vi "SetAngles.vi"(8 "error in (no error)":errorcluster, 10 "Angles":T1, 11 "reference in":refnum<class "Manipulator.lvclass">) -> (0 "error out":errorcluster, 3 "reference out":refnum<class "Manipulator.lvclass">)   [LabVIEW 2014, in "Manipulator.lvclass"]
uses:
  Manipulator.lvclass
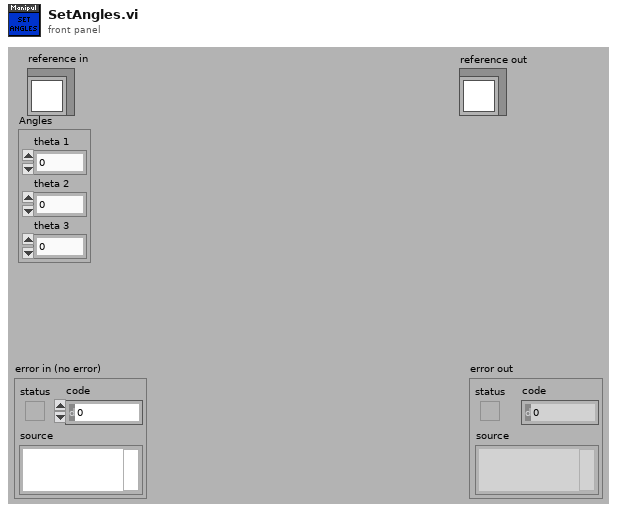
[diagram p1: front panel]
types:
  T1 = cluster{"theta 1":dbl, "theta 2":dbl, "theta 3":dbl}
  T2 = typedef "Manipulator.lvclass/ObjectAttributes.ctl" = cluster{"Coordinates":cluster{"X":dbl, "Y":dbl, "Z":dbl}, "Angles":cluster{"THETA_1":dbl, "THETA_2":dbl, "THETA_3":dbl, "THETA_4":dbl, "THETA_5":dbl, "THETA_6":dbl, "THETA_7":dbl, "THETA_8":dbl, "THETA_9":dbl, "THETA_10":dbl}, "Lengths":cluster{"a":dbl, "b":dbl, "c":dbl, "d":dbl, "e":dbl}, "Coordinates of joints":cluster{"A":cluster{"X":dbl, "Y":dbl, "Z":dbl}, "B":cluster{"X":dbl, "Y":dbl, "Z":dbl}, "C":cluster{"X":dbl, "Y":dbl, "Z":dbl}, "D":cluster{"X":dbl, "Y":dbl, "Z":dbl}}}
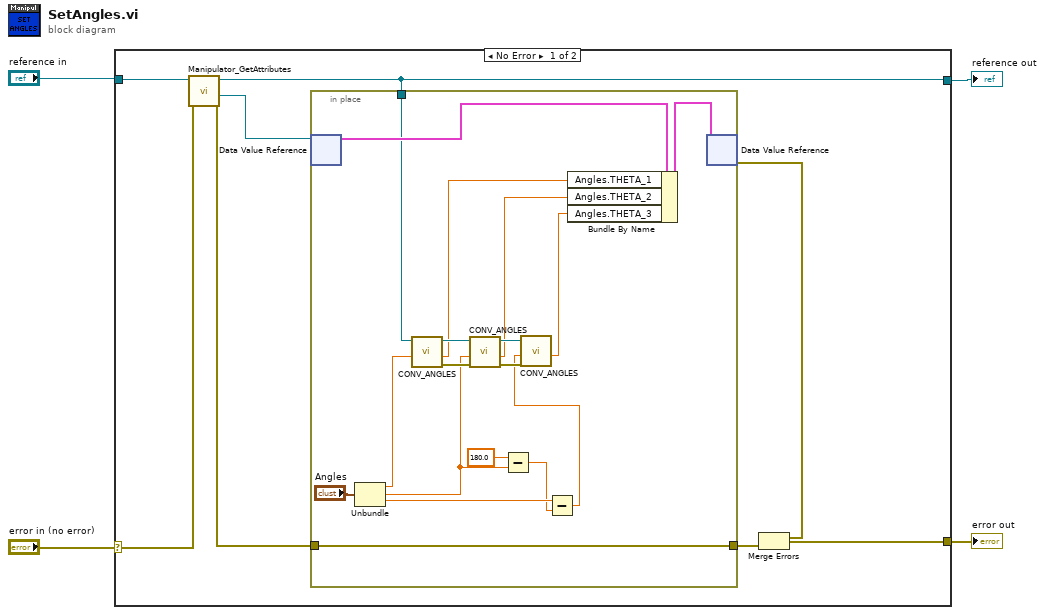
[diagram p0: block diagram]
diagram:
  n1 = case shown="No Error" "error in (no error)" {
    selector: "error in (no error)" -> [w9 w32]
    tunnel: [w11 w32] -> w3
    tunnel: [w5 w31] -> w1
    tunnel: "reference in" -> [w10 w31]
    frame No Error {
      n2 = call "Manipulator_GetAttributes.vi"("error in (no error)"=w9, "reference in"=w10) -> ("error out"=w8:errorcluster, "DataRef"=w6:refnum<data-value>, "reference out"=w5:refnum<class "Manipulator.lvclass">)  [unwired: 6 in, 1 out]
      n3 = in-place {
        in-place-border: w8 -> [w29]
        in-place-border: [w29] -> w7
        in-place-border: w5 -> [w26]
        n4 = in-place-dvr #1(w6) -> (w28:T2)  [unwired: 1 out]
        n5 = Unbundle("Angles") -> ("theta 1"=w21:dbl, "theta 2"=w14:dbl, "theta 3"=w16:dbl)
        n6 = call "CONV_ANGLES.vi"("IN (DEG)"=w21, "reference in"=w26) -> ("error out"=w25:errorcluster, "OUT (RAD)"=w20:dbl, "reference out"=w24:refnum<class "Manipulator.lvclass">)  [unwired: 6 in, 1 out]
        n7 = call "CONV_ANGLES.vi"("error in (no error)"=w25, "IN (DEG)"=w14, "reference in"=w24) -> ("error out"=w23:errorcluster, "OUT (RAD)"=w19:dbl, "reference out"=w22:refnum<class "Manipulator.lvclass">)  [unwired: 5 in, 1 out]
        n8 = Subtract(x=180.0, y=w14) -> (x-y=w15:dbl)
        n9 = Subtract(x=w16, y=w15) -> (x-y=w13:dbl)
        n10 = call "CONV_ANGLES.vi"("error in (no error)"=w23, "IN (DEG)"=w13, "reference in"=w22) -> ("OUT (RAD)"=w18:dbl)  [unwired: 5 in, 3 out]
        n11 = Bundle By Name(cluster=w28, "Angles.THETA_1"=w20, "Angles.THETA_2"=w19, "Angles.THETA_3"=w18) -> (w30:T2)
        n12 = in-place-dvr #1(w30) -> (w12:errorcluster)  [unwired: 1 out]
      }
      n13 = Merge Errors(w12, w7) -> (w11:errorcluster)
    }
    frame Error {
    }
  }
  "error out" <- w3
  "reference out" <- w1
